vi "Decorator.vi"(10 "Actor":refnum<class "Actor.lvclass">, 11 "Ex Queue Actor in":refnum<class "Ex Queue Actor.lvclass">) -> (3 "Ex Queue Actor out":refnum<class "Ex Queue Actor.lvclass">)   [LabVIEW 2021, in "Ex Queue Actor.lvlib" / "Ex Queue Actor.lvclass"]
uses:
  Ex Queue Actor.lvclass
  Actor/Actor/Actor.lvclass
  Actor/Queue Actor/Queue Actor.lvclass
  Ex Queue Actor.lvclass/Ex Queue Actor.ctl
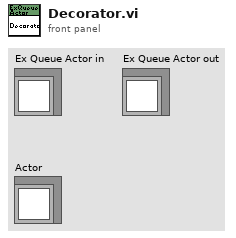
[diagram p1: front panel]
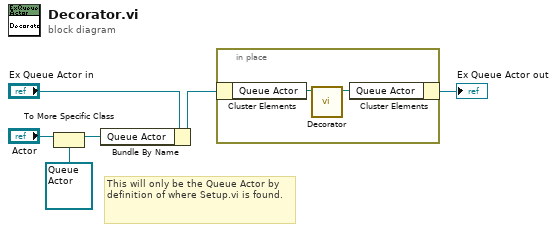
[diagram p0: block diagram]
diagram:
  # "This will only be the Queue Actor by definition of where Setup.vi is found."
  n1 = To More Specific Class(target class=refnum<class "Queue Actor.lvclass"> refnum ("Queue Actor"), reference="Actor") -> (specific class reference=w3:refnum<class "Queue Actor.lvclass">)  [unwired: 1 in, 1 out]
  n2 = Bundle By Name(cluster="Ex Queue Actor in", "Queue Actor"=w3) -> (w5:refnum<class "Ex Queue Actor.lvclass">)
  n3 = in-place {
    n4 = in-place-cluster #1(w5) -> ("Queue Actor"=w8:refnum<class "Queue Actor.lvclass">)
    n5 = call-dynamic "Decorator.vi"("Actor in"=w8) -> ("Actor out"=w7:refnum<class "Queue Actor.lvclass">)  [unwired: 10 in]
    n6 = in-place-cluster #1("Queue Actor"=w7) -> (→"Ex Queue Actor out":refnum<class "Ex Queue Actor.lvclass">)
  }
